vi "rszvl_core_global.vi"() -> ()   [LabVIEW 2014] (continued)
"Restricted Repeated Capabilities"="", "Help"="This attribute switches on and off the calibration info in the custom header. The custom header can be added to an exported trace file.\n\nAvailable Repeated Capabilities:\nNone\n\nRemote-control command(s):\nMMEMory:STORe:TRACe:USER:CINFo ON | OFF", "Flags"={"OPC Wait"=FALSE, "Dont check status"=FALSE, "*WAI"=FALSE}, "Check Status Callback"=""}, {"Level"=1, "Descriptive Name"="NWA Markers", "Class Only"=TRUE, "Data Type"=0, "Access"=0, "Identifier"="", "Range Table"="", "Command"="", "Read Callback"="", "Write Callback"="", "Range Callback"="", "Check Callback"="", "Rngtable Callback"="", "Coerce Callback"="", "User Callback"="", "Supported Models"="", "Instrument Options"="", "Repeated Capabilities"="", "Restricted Repeated Capabilities"="", "Help"="(1) NWA Marker State:\nThis attribute creates the marker numbered <Mk> and assigns it to trace no. <Chn>.\n\n(2) NWA Marker Stimulus:\nThis attribute defines the stimulus (in Cartesian diagrams: x-axis) value of the marker no. <Mk>, which can (but doesn't have to) be created using CALCulate<Chn>:MARKer<Mk>[:STATe] ON (attribute RSZVL_ATTR_NWA_MARKER_STATE).\n\n(3) NWA Marker Reference State:\nThis attribute creates the reference marker and assigns it to trace no. <Chn>.\n\n(4) NWA Marker Reference Stimulus:\nThis attribute defines the stimulus (in Cartesian diagrams: x-axis) value of the reference marker, which can (but doesn't have to) be displayed using CALCulate<Chn>:MARKer<Mk>:REFerence[:STATe] ON (attribute RSZVL_ATTR_NWA_MARKER_STATE). \n\n(5) NWA Delta Marker State:\nThis attribute switches the delta mode for marker <Mk> on trace no. <Chn> on or off. The marker must be created before using CALCulate<Chn>:MARKer<Mk>[:STATe] ON (attribute RSZVL_ATTR_NWA_MARKER_STATE). If the active trace contains no reference marker, the command also creates a reference marker.\n\n(6) NWA Marker Coupled:\nThis attribute couples the markers of all traces in the active setup to the markers of trace no. <Chn>, provided that they have the same sweep type (SENSe<Chn>:FUNCtion).\n\n(7) NWA Marker Mode:\nThis attribute sets marker no. <Mk> to continuous or discrete mode. The marker doesn't have to be created before (CALCulate<Chn>:MARKer<Mk>[:STATe] ON), the mode can be assigned in advance.\n\n(8) NWA Marker Fixed:\nThis attribute sets marker no. <Mk> to normal or fixed mode. The marker must be created before using CALCulate<Ch/Tr>:MARKer<Mk>[:STATe] ON (attribute RSZVL_ATTR_NWA_MARKER_STATE). \n\n(9) NWA Marker Search Tracking:\nThis attribute enables or disables the marker tracking mode for marker no. <Mk>. Tracking mode causes the active minimum/maximum or target search of the active marker to be repeated after each sweep. A marker must be created and a search mode must be active (CALCulate<Chn>:MARKer<Mk>:FUNCtion:EXECute ...) to use this attribute.\n\n(10) NWA All Markers Off:\nThis attribute removes all markers from all traces of the active setup. The removed markers remember their properties (stimulus value, format, delta mode, number) when they are restored (CALC<Chn>:MARK<Mk> ON). The marker properties are definitely lost if the associated trace is deleted. \n\n(11) NWA Marker To Center:\nThis attribute sets the center of the sweep range equal to the stimulus value of the marker <Mk> on trace no. <Chn>.\n\n(12) NWA Marker To Start Frequency:\nThis attribute sets the beginning (start) of the sweep range equal to the stimulus value of the marker <Mk> on trace no. <Chn>.\n\n(13) NWA Marker To Stop Frequency:\nThis attribute sets the end (stop) of the sweep range equal to the stimulus value of the marker <Mk> on trace no. <Chn>.\n\n(14) NWA Marker Format:\nThis attribute defines the output format for the (complex) value of marker <Mk> on trace no. <Chn>.\n\n(15) NWA Marker Search:\nThis attribute selects a search mode for marker no. <Mk> and initiates the search. The marker must be created before using CALCulate<Chn>:MARKer<Mk>[:STATe] ON (exception: bandfilter search). \n\n(16) NWA Marker Bandfilter Search Mode:\nThis attribute selects the bandfilter search mode.\n\n(17) NWA Marker Search Range:\nThis attribute assigns a search range no. <numeric_value> to marker no <Mk> and selects the search range, e.g. in order to define the start and stop values.\n\n(18) NWA Marker Search Range Start:\nThis attribute defines the start value of the search range selected with CALCulate<Chn>:MARKer<Mk>:FUNCtion:DOMain:USER (attribute RSZVL_ATTR_NWA_MARKER_SEARCH_RANGE). \n\n(19) NWA Marker Search Range Stop:\nThis attribute defines the stop value of the search range selected with CALCulate<Chn>:MARKer<Mk>:FUNCtion:DOMain:USER (attribute RSZVL_ATTR_NWA_MARKER_SEARCH_RANGE). \n\n(20) NWA Marker Target Value:\nThis attribute defines the target value for the target search of marker no. <Mk>, which can be activated using CALCulate<Chn>:MARKer<Mk>:FUCTion:EXECute TARGet (attribute RSZVL_ATTR_NWA_MARKER_SEARCH_MODE). \n\n(21) NWA Marker Bandwidth:\nThis attribute sets the bandfilter level for a bandfilter search or returns the results. The attribute is only available after a bandfilter search has been executed (CALCulate<Chn>:MARKer<Mk>:FUNCtion:EXECute BFILter).\n\n(22) NWA Marker Show Bandfilter Search Results:\nThis attribute shows or hides the bandfilter search results in the diagram area.\n\n(23) NWA Save All Markers:\nThis attribute saves the values of all markers to a ASCII file.", "Flags"={"OPC Wait"=FALSE, "Dont check status"=FALSE, "*WAI"=FALSE}, "Check Status Callback"=""}, {"Level"=2, "Descriptive Name"="NWA Marker State", "Class Only"=FALSE, "Data Type"=3, "Access"=2, "Identifier"="RSZVL_ATTR_NWA_MARKER_STATE", "Range Table"="", "Command"="CALC{Channel}:MARK{NWAMarker}:STAT", "Read Callback"="", "Write Callback"="", "Range Callback"="", "Check Callback"="", "Rngtable Callback"="", "Coerce Callback"="", "User Callback"="", "Supported Models"="", "Instrument Options"="", "Repeated Capabilities"="", "Restricted Repeated Capabilities"="", "Help"="This attribute creates the marker numbered <Mk> and assigns it to trace no. <Chn>.\n\nAvailable Repeated Capabilities:\nChannel: CH1,CH2,CH3,CH4,CH5,CH6,CH7,CH8,CH9,CH10,CH11,CH12,CH13,CH14,CH15,CH16,CH17,CH18,CH19,CH20\r\nNWAMarker: MAR1,MAR2,MAR3,MAR4,MAR5,MAR6,MAR7,MAR8,MAR9,MAR10\r\n\nRemote-control command(s):\nCALCulate<Chn>:MARKer<Mk>[:STATe] ON | OFF", "Flags"={"OPC Wait"=FALSE, "Dont check status"=FALSE, "*WAI"=FALSE}, "Check Status Callback"=""}, {"Level"=2, "Descriptive Name"="NWA Marker Stimulus", "Class Only"=FALSE, "Data Type"=1, "Access"=2, "Identifier"="RSZVL_ATTR_NWA_MARKER_X", "Range Table"="rszvl_rngNWAMarkerStimulus", "Command"="CALC{Channel}:MARK{NWAMarker}:X", "Read Callback"="", "Write Callback"="", "Range Callback"="", "Check Callback"="", "Rngtable Callback"="", "Coerce Callback"="", "User Callback"="", "Supported Models"="", "Instrument Options"="", "Repeated Capabilities"="", "Restricted Repeated Capabilities"="", "Help"="This attribute defines the stimulus (in Cartesian diagrams: x-axis) value of the marker no. <Mk>, which can (but doesn't have to) be created using CALCulate<Chn>:MARKer<Mk>[:STATe] ON (attribute RSZVL_ATTR_NWA_MARKER_STATE).\n\nAvailable Repeated Capabilities:\nChannel: CH1,CH2,CH3,CH4,CH5,CH6,CH7,CH8,CH9,CH10,CH11,CH12,CH13,CH14,CH15,CH16,CH17,CH18,CH19,CH20\r\nNWAMarker: MAR1,MAR2,MAR3,MAR4,MAR5,MAR6,MAR7,MAR8,MAR9,MAR10\r\n\nRemote-control command(s):\nCALCulate<Chn>:MARKer<Mk>:X", "Flags"={"OPC Wait"=FALSE, "Dont check status"=FALSE, "*WAI"=FALSE}, "Check Status Callback"=""}, {"Level"=2, "Descriptive Name"="NWA Marker Reference State", "Class Only"=FALSE, "Data Type"=3, "Access"=2, "Identifier"="RSZVL_ATTR_NWA_MARKER_REF_STATE", "Range Table"="", "Command"="CALC{Channel}:MARK{NWAMarker}:REF:STAT", "Read Callback"="", "Write Callback"="", "Range Callback"="", "Check Callback"="", "Rngtable Callback"="", "Coerce Callback"="", "User Callback"="", "Supported Models"="", "Instrument Options"="", "Repeated Capabilities"="", "Restricted Repeated Capabilities"="", "Help"="This attribute creates the reference marker and assigns it to trace no. <Chn>.\n\nAvailable Repeated Capabilities:\nChannel: CH1,CH2,CH3,CH4,CH5,CH6,CH7,CH8,CH9,CH10,CH11,CH12,CH13,CH14,CH15,CH16,CH17,CH18,CH19,CH20\r\nNWAMarker: MAR1,MAR2,MAR3,MAR4,MAR5,MAR6,MAR7,MAR8,MAR9,MAR10\r\n\nRemote-control command(s):\nCALCulate<Chn>:MARKer<Mk>:REFerence[:STATe] ON | OFF", "Flags"={"OPC Wait"=FALSE, "Dont check status"=FALSE, "*WAI"=FALSE}, "Check Status Callback"=""}, {"Level"=2, "Descriptive Name"="NWA Marker Reference Stimulus", "Class Only"=FALSE, "Data Type"=1, "Access"=2, "Identifier"="RSZVL_ATTR_NWA_MARKER_REF_X", "Range Table"="rszvl_rngNWAMarkerStimulus", "Command"="CALC{Channel}:MARK{NWAMarker}:REF:X", "Read Callback"="", "Write Callback"="", "Range Callback"="", "Check Callback"="", "Rngtable Callback"="", "Coerce Callback"="", "User Callback"="", "Supported Models"="", "Instrument Options"="", "Repeated Capabilities"="", "Restricted Repeated Capabilities"="", "Help"="This attribute defines the stimulus (in Cartesian diagrams: x-axis) value of the reference marker, which can (but doesn't have to) be displayed using CALCulate<Chn>:MARKer<Mk>:REFerence[:STATe] ON (attribute RSZVL_ATTR_NWA_MARKER_STATE).\n\nAvailable Repeated Capabilities:\nChannel: CH1,CH2,CH3,CH4,CH5,CH6,CH7,CH8,CH9,CH10,CH11,CH12,CH13,CH14,CH15,CH16,CH17,CH18,CH19,CH20\r\nNWAMarker: MAR1,MAR2,MAR3,MAR4,MAR5,MAR6,MAR7,MAR8,MAR9,MAR10\r\n\nRemote-control command(s):\nCALCulate<Chn>:MARKer<Mk>:REFerence:X", "Flags"={"OPC Wait"=FALSE, "Dont check status"=FALSE, "*WAI"=FALSE}, "Check Status Callback"=""}, {"Level"=2, "Descriptive Name"="NWA Marker Reference Mode", "Class Only"=FALSE, "Data Type"=0, "Access"=2, "Identifier"="RSZVL_ATTR_NWA_MARKER_REF_MODE", "Range Table"="rszvl_rngNWAMarkerMode", "Command"="CALC{Channel}:MARK{NWAMarker}:REF:MODE", "Read Callback"="", "Write Callback"="", "Range Callback"="", "Check Callback"="", "Rngtable Callback"="", "Coerce Callback"="", "User Callback"="", "Supported Models"="", "Instrument Options"="", "Repeated Capabilities"="", "Restricted Repeated Capabilities"="", "Help"="This attribute sets the reference marker to continuous or discrete mode. The marker doesn't have to be created before\n(CALCulate<Chn>:MARKer<Mk>:REFerence[:STATe] ON), the mode can be assigned in advance.\n\nAvailable Repeated Capabilities:\nChannel: CH1,CH2,CH3,CH4,CH5,CH6,CH7,CH8,CH9,CH10,CH11,CH12,CH13,CH14,CH15,CH16,CH17,CH18,CH19,CH20\r\nNWAMarker: MAR1,MAR2,MAR3,MAR4,MAR5,MAR6,MAR7,MAR8,MAR9,MAR10\r\n\nRemote-control command(s):\nCALCulate<Chn>:MARKer<Mk>:REFerence:MODE CONTinuous | DISCrete", "Flags"={"OPC Wait"=FALSE, "Dont check status"=FALSE, "*WAI"=FALSE}, "Check Status Callback"=""}, {"Level"=2, "Descriptive Name"="NWA Marker Referece Fixed", "Class Only"=FALSE, "Data Type"=0, "Access"=2, "Identifier"="RSZVL_ATTR_NWA_MARKER_REF_FIXED", "Range Table"="rszvl_rngNWAMarkerType", "Command"="CALC{Channel}:MARK{NWAMarker}:REF:TYPE", "Read Callback"="", "Write Callback"="", "Range Callback"="", "Check Callback"="", "Rngtable Callback"="", "Coerce Callback"="", "User Callback"="", "Supported Models"="", "Instrument Options"="", "Repeated Capabilities"="", "Restricted Repeated Capabilities"="", "Help"="This attribute sets the reference to normal or fixed mode. The marker must be created before using\nCALCulate<Chn>:MARKer<Mk>:REFerence[:STATe] ON.\n\nAvailable Repeated Capabilities:\nChannel: CH1,CH2,CH3,CH4,CH5,CH6,CH7,CH8,CH9,CH10,CH11,CH12,CH13,CH14,CH15,CH16,CH17,CH18,CH19,CH20\r\nNWAMarker: MAR1,MAR2,MAR3,MAR4,MAR5,MAR6,MAR7,MAR8,MAR9,MAR10\r\n\nRemote-control command(s):\nCALCulate<Chn>:MARKer<Mk>:REFerence:TYPE NORMal | FIXed", "Flags"={"OPC Wait"=FALSE, "Dont check status"=FALSE, "*WAI"=FALSE}, "Check Status Callback"=""}, {"Level"=2, "Descriptive Name"="NWA Delta Marker State", "Class Only"=FALSE, "Data Type"=3, "Access"=2, "Identifier"="RSZVL_ATTR_NWA_DELTA_MARKER_STATE", "Range Table"="", "Command"="CALC{Channel}:MARK{NWAMarker}:DELT:STAT", "Read Callback"="", "Write Callback"="", "Range Callback"="", "Check Callback"="", "Rngtable Callback"="", "Coerce Callback"="", "User Callback"="", "Supported Models"="", "Instrument Options"="", "Repeated Capabilities"="", "Restricted Repeated Capabilities"="", "Help"="This attribute switches the delta mode for marker <Mk> on trace no. <Chn> on or off. The marker must be created before using CALCulate<Chn>:MARKer<Mk>[:STATe] ON (attribute RSZVL_ATTR_NWA_MARKER_STATE). If the active trace contains no reference marker, the command also creates a reference marker.\n\nAvailable Repeated Capabilities:\nChannel: CH1,CH2,CH3,CH4,CH5,CH6,CH7,CH8,CH9,CH10,CH11,CH12,CH13,CH14,CH15,CH16,CH17,CH18,CH19,CH20\r\nNWAMarker: MAR1,MAR2,MAR3,MAR4,MAR5,MAR6,MAR7,MAR8,MAR9,MAR10\r\n\nRemote-control command(s):\nCALCulate<Chn>:MARKer<Mk>:DELTa[:STATe] ON | OFF", "Flags"={"OPC Wait"=FALSE, "Dont check status"=FALSE, "*WAI"=FALSE}, "Check Status Callback"=""}, {"Level"=2, "Descriptive Name"="NWA Marker Coupled", "Class Only"=FALSE, "Data Type"=3, "Access"=2, "Identifier"="RSZVL_ATTR_NWA_MARKER_COUPLED", "Range Table"="", "Command"="CALC{Channel}:MARK:COUP:STAT", "Read Callback"="", "Write Callback"="", "Range Callback"="", "Check Callback"="", "Rngtable Callback"="", "Coerce Callback"="", "User Callback"="", "Supported Models"="", "Instrument Options"="", "Repeated Capabilities"="", "Restricted Repeated Capabilities"="", "Help"="This attribute couples the markers of all traces in the active setup to the markers of trace no. <Chn>, provided that they have the same sweep type (SENSe<Chn>:FUNCtion).\n\nAvailable Repeated Capabilities:\nChannel: CH1,CH2,CH3,CH4,CH5,CH6,CH7,CH8,CH9,CH10,CH11,CH12,CH13,CH14,CH15,CH16,CH17,CH18,CH19,CH20\r\n\nRemote-control command(s):\nCALCulate<Chn>:MARKer<Mk>:COUPled[:STATe] ON | OFF", "Flags"={"OPC Wait"=FALSE, "Dont check status"=FALSE, "*WAI"=FALSE}, "Check Status Callback"=""}, {"Level"=2, "Descriptive Name"="NWA Marker Mode", "Class Only"=FALSE, "Data Type"=0, "Access"=2, "Identifier"="RSZVL_ATTR_NWA_MARKER_MODE", "Range Table"="rszvl_rngNWAMarkerMode", "Command"="CALC{Channel}:MARK{NWAMarker}:MODE", "Read Callback"="", "Write Callback"="", "Range Callback"="", "Check Callback"="", "Rngtable Callback"="", "Coerce Callback"="", "User Callback"="", "Supported Models"="", "Instrument Options"="", "Repeated Capabilities"="", "Restricted Repeated Capabilities"="", "Help"="This attribute sets marker no. <Mk> to continuous or discrete mode. The marker doesn't have to be created before (CALCulate<Chn>:MARKer<Mk>[:STATe] ON), the mode can be assigned in advance.\n\nAvailable Repeated Capabilities:\nChannel: CH1,CH2,CH3,CH4,CH5,CH6,CH7,CH8,CH9,CH10,CH11,CH12,CH13,CH14,CH15,CH16,CH17,CH18,CH19,CH20\r\nNWAMarker: MAR1,MAR2,MAR3,MAR4,MAR5,MAR6,MAR7,MAR8,MAR9,MAR10\r\n\nRemote-control command(s):\nCALCulate<Chn>:MARKer<Mk>:MODE CONTinuous | DISCrete", "Flags"={"OPC Wait"=FALSE, "Dont check status"=FALSE, "*WAI"=FALSE}, "Check Status Callback"=""}, {"Level"=2, "Descriptive Name"="NWA Marker Fixed", "Class Only"=FALSE, "Data Type"=0, "Access"=2, "Identifier"="RSZVL_ATTR_NWA_MARKER_TYPE", "Range Table"="rszvl_rngNWAMarkerType", "Command"="CALC{Channel}:MARK{NWAMarker}:TYPE", "Read Callback"="", "Write Callback"="", "Range Callback"="", "Check Callback"="", "Rngtable Callback"="", "Coerce Callback"="", "User Callback"="", "Supported Models"="", "Instrument Options"="", "Repeated Capabilities"="", "Restricted Repeated Capabilities"="", "Help"="This attribute sets marker no. <Mk> to normal or fixed mode. The marker must be created before using CALCulate<Ch/Tr>:MARKer<Mk>[:STATe] ON (attribute RSZVL_ATTR_NWA_MARKER_STATE).\n\nAvailable Repeated Capabilities:\nChannel: CH1,CH2,CH3,CH4,CH5,CH6,CH7,CH8,CH9,CH10,CH11,CH12,CH13,CH14,CH15,CH16,CH17,CH18,CH19,CH20\r\nNWAMarker: MAR1,MAR2,MAR3,MAR4,MAR5,MAR6,MAR7,MAR8,MAR9,MAR10\r\n\nRemote-control command(s):\nCALCulate<Chn>:MARKer<Mk>:TYPE NORMal | FIXed", "Flags"={"OPC Wait"=FALSE, "Dont check status"=FALSE, "*WAI"=FALSE}, "Check Status Callback"=""}, {"Level"=2, "Descriptive Name"="NWA Marker Search Tracking", "Class Only"=FALSE, "Data Type"=3, "Access"=2, "Identifier"="RSZVL_ATTR_NWA_MARKER_SEARCH_TRACKING", "Range Table"="", "Command"="CALC{Channel}:MARK{NWAMarker}:SEAR:TRAC", "Read Callback"="", "Write Callback"="", "Range Callback"="", "Check Callback"="", "Rngtable Callback"="", "Coerce Callback"="", "User Callback"="", "Supported Models"="", "Instrument Options"="", "Repeated Capabilities"="", "Restricted Repeated Capabilities"="", "Help"="This attribute enables or disables the marker tracking mode for marker no. <Mk>. Tracking mode causes the active minimum/maximum or target search of the active marker to be repeated after each sweep. A marker must be created and a search mode must be active (CALCulate<Chn>:MARKer<Mk>:FUNCtion:EXECute ...) to use this attribute.\n\nAvailable Repeated Capabilities:\nChannel: CH1,CH2,CH3,CH4,CH5,CH6,CH7,CH8,CH9,CH10,CH11,CH12,CH13,CH14,CH15,CH16,CH17,CH18,CH19,CH20\r\nNWAMarker: MAR1,MAR2,MAR3,MAR4,MAR5,MAR6,MAR7,MAR8,MAR9,MAR10\r\n\nRemote-control command(s):\nCALCulate<Chn>:MARKer<Mk>:SEARch:TRACking ON | OFF", "Flags"={"OPC Wait"=FALSE, "Dont check status"=FALSE, "*WAI"=FALSE}, "Check Status Callback"=""}, {"Level"=2, "Descriptive Name"="NWA All Markers Off", "Class Only"=FALSE, "Data Type"=4, "Access"=1, "Identifier"="RSZVL_ATTR_NWA_MARKER_AOFF", "Range Table"="", "Command"="CALC{Channel}:MARK:AOFF", "Read Callback"="", "Write Callback"="", "Range Callback"="", "Check Callback"="", "Rngtable Callback"="", "Coerce Callback"="", "User Callback"="", "Supported Models"="", "Instrument Options"="", "Repeated Capabilities"="", "Restricted Repeated Capabilities"="", "Help"="This attribute removes all markers from all traces of the active setup. The removed markers remember their properties (stimulus value, format, delta mode, number) when they are restored (CALC<Chn>:MARK<Mk> ON). The marker properties are definitely lost if the associated trace is deleted.\n\nAvailable Repeated Capabilities:\nChannel: CH1,CH2,CH3,CH4,CH5,CH6,CH7,CH8,CH9,CH10,CH11,CH12,CH13,CH14,CH15,CH16,CH17,CH18,CH19,CH20\r\n\nRemote-control command(s):\nCALCulate<Chn>:MARKer<Mk>:AOFF", "Flags"={"OPC Wait"=FALSE, "Dont check status"=FALSE, "*WAI"=FALSE}, "Check Status Callback"=""}, {"Level"=2, "Descriptive Name"="NWA Marker To Center", "Class Only"=FALSE, "Data Type"=4, "Access"=1, "Identifier"="RSZVL_ATTR_NWA_MARKER_TO_CENTER", "Range Table"="", "Command"="CALC{Channel}:MARK{NWAMarker}:FUNC:CENT", "Read Callback"="", "Write Callback"="", "Range Callback"="", "Check Callback"="", "Rngtable Callback"="", "Coerce Callback"="", "User Callback"="", "Supported Models"="", "Instrument Options"="", "Repeated Capabilities"="", "Restricted Repeated Capabilities"="", "Help"="This attribute sets the center of the sweep range equal to the stimulus value of the marker <Mk> on trace no. <Chn>.\n\nAvailable Repeated Capabilities:\nChannel: CH1,CH2,CH3,CH4,CH5,CH6,CH7,CH8,CH9,CH10,CH11,CH12,CH13,CH14,CH15,CH16,CH17,CH18,CH19,CH20\r\nNWAMarker: MAR1,MAR2,MAR3,MAR4,MAR5,MAR6,MAR7,MAR8,MAR9,MAR10\r\n\nRemote-control command(s):\nCALCulate<Chn>:MARKer<Mk>:FUNCtion:CENTer", "Flags"={"OPC Wait"=FALSE, "Dont check status"=FALSE, "*WAI"=FALSE}, "Check Status Callback"=""}, {"Level"=2, "Descriptive Name"="NWA Marker To Start Frequency", "Class Only"=FALSE, "Data Type"=4, "Access"=1, "Identifier"="RSZVL_ATTR_NWA_MARKER_TO_START", "Range Table"="", "Command"="CALC{Channel}:MARK{NWAMarker}:FUNC:STAR", "Read Callback"="", "Write Callback"="", "Range Callback"="", "Check Callback"="", "Rngtable Callback"="", "Coerce Callback"="", "User Callback"="", "Supported Models"="", "Instrument Options"="", "Repeated Capabilities"="", "Restricted Repeated Capabilities"="", "Help"="This attribute sets the beginning (start) of the sweep range equal to the stimulus value of the marker <Mk> on trace no. <Chn>.\n\nAvailable Repeated Capabilities:\nChannel: CH1,CH2,CH3,CH4,CH5,CH6,CH7,CH8,CH9,CH10,CH11,CH12,CH13,CH14,CH15,CH16,CH17,CH18,CH19,CH20\r\nNWAMarker: MAR1,MAR2,MAR3,MAR4,MAR5,MAR6,MAR7,MAR8,MAR9,MAR10\r\n\nRemote-control command(s):\nCALCulate<Chn>:MARKer<Mk>:FUNCtion:STARt", "Flags"={"OPC Wait"=FALSE, "Dont check status"=FALSE, "*WAI"=FALSE}, "Check Status Callback"=""}, {"Level"=2, "Descriptive Name"="NWA Marker To Stop Frequency", "Class Only"=FALSE, "Data Type"=4, "Access"=1, "Identifier"="RSZVL_ATTR_NWA_MARKER_TO_STOP", "Range Table"="", "Command"="CALC{Channel}:MARK{NWAMarker}:FUNC:STOP", "Read Callback"="", "Write Callback"="", "Range Callback"="", "Check Callback"="", "Rngtable Callback"="", "Coerce Callback"="", "User Callback"="", "Supported Models"="", "Instrument Options"="", "Repeated Capabilities"="", "Restricted Repeated Capabilities"="", "Help"="This attribute sets the end (stop) of the sweep range equal to the stimulus value of the marker <Mk> on trace no. <Chn>.\n\nAvailable Repeated Capabilities:\nChannel: CH1,CH2,CH3,CH4,CH5,CH6,CH7,CH8,CH9,CH10,CH11,CH12,CH13,CH14,CH15,CH16,CH17,CH18,CH19,CH20\r\nNWAMarker: MAR1,MAR2,MAR3,MAR4,MAR5,MAR6,MAR7,MAR8,MAR9,MAR10\r\n\nRemote-control command(s):\nCALCulate<Chn>:MARKer<Mk>:FUNCtion:STOP", "Flags"={"OPC Wait"=FALSE, "Dont check status"=FALSE, "*WAI"=FALSE}, "Check Status Callback"=""}, {"Level"=2, "Descriptive Name"="NWA Marker Format", "Class Only"=FALSE, "Data Type"=0, "Access"=2, "Identifier"="RSZVL_ATTR_NWA_MARKER_FORMAT", "Range Table"="rszvl_rngNWAMarkerFormat", "Command"="CALC{Channel}:MARK{NWAMarker}:FORM", "Read Callback"="", "Write Callback"="", "Range Callback"="", "Check Callback"="", "Rngtable Callback"="", "Coerce Callback"="", "User Callback"="", "Supported Models"="", "Instrument Options"="", "Repeated Capabilities"="", "Restricted Repeated Capabilities"="", "Help"="This attribute defines the output format for the (complex) value of marker <Mk> on trace no. <Chn>.\n\nAvailable Repeated Capabilities:\nChannel: CH1,CH2,CH3,CH4,CH5,CH6,CH7,CH8,CH9,CH10,CH11,CH12,CH13,CH14,CH15,CH16,CH17,CH18,CH19,CH20\r\nNWAMarker: MAR1,MAR2,MAR3,MAR4,MAR5,MAR6,MAR7,MAR8,MAR9,MAR10\r\n\nRemote-control command(s):\nCALCulate<Chn>:MARKer<Mk>:FORMat MLINear | MLOGarithmic | PHASe | POLar | GDELay | REAL | IMAGinary | SWR | LINPhase | LOGPhase | IMPedance | ADMittance", "Flags"={"OPC Wait"=FALSE, "Dont check status"=FALSE, "*WAI"=FALSE}, "Check Status Callback"=""}, {"Level"=2, "Descriptive Name"="NWA Marker Search", "Class Only"=FALSE, "Data Type"=0, "Access"=1, "Identifier"="RSZVL_ATTR_NWA_MARKER_SEARCH_MODE", "Range Table"="rszvl_rngNWAMarkerSearch", "Command"="CALC{Channel}:MARK{NWAMarker}:FUNC:EXEC", "Read Callback"="", "Write Callback"="", "Range Callback"="", "Check Callback"="", "Rngtable Callback"="", "Coerce Callback"="", "User Callback"="", "Supported Models"="", "Instrument Options"="", "Repeated Capabilities"="", "Restricted Repeated Capabilities"="", "Help"="This attribute selects a search mode for marker no. <Mk> and initiates the search. The marker must be created before using CALCulate<Chn>:MARKer<Mk>[:STATe] ON (exception: bandfilter search).\n\nAvailable Repeated Capabilities:\nChannel: CH1,CH2,CH3,CH4,CH5,CH6,CH7,CH8,CH9,CH10,CH11,CH12,CH13,CH14,CH15,CH16,CH17,CH18,CH19,CH20\r\nNWAMarker: MAR1,MAR2,MAR3,MAR4,MAR5,MAR6,MAR7,MAR8,MAR9,MAR10\r\n\nRemote-control command(s):\nCALCulate<Chn>:MARKer<Mk>:FUNCtion:EXECute MAXimum | MINimum | RPEak | LPEak | NPEak | TARGet | LTARget | RTARget | BFILter", "Flags"={"OPC Wait"=FALSE, "Dont check status"=FALSE, "*WAI"=FALSE}, "Check Status Callback"=""}, {"Level"=2, "Descriptive Name"="NWA Marker Bandfilter Search Mode", "Class Only"=FALSE, "Data Type"=0, "Access"=2, "Identifier"="RSZVL_ATTR_NWA_MARKER_BFILTER_SEARCH_MODE", "Range Table"="rszvl_rngNWAMarkerBFilterSearchMode", "Command"="CALC{Channel}:MARK:FUNC:BWID:MODE", "Read Callback"="", "Write Callback"="", "Range Callback"="", "Check Callback"="", "Rngtable Callback"="", "Coerce Callback"="", "User Callback"="", "Supported Models"="", "Instrument Options"="", "Repeated Capabilities"="", "Restricted Repeated Capabilities"="", "Help"="This attribute selects the bandfilter search mode.\n\nAvailable Repeated Capabilities:\nChannel: CH1,CH2,CH3,CH4,CH5,CH6,CH7,CH8,CH9,CH10,CH11,CH12,CH13,CH14,CH15,CH16,CH17,CH18,CH19,CH20\r\n\nRemote-control command(s):\nCALCulate<Chn>:MARKer<Mk>:FUNCtion:BWIDth:MODE BPASs | BSTop | BPRMarker | BSRMarker", "Flags"={"OPC Wait"=FALSE, "Dont check status"=FALSE, "*WAI"=FALSE}, "Check Status Callback"=""}, {"Level"=2, "Descriptive Name"="NWA Marker Search Range", "Class Only"=FALSE, "Data Type"=0, "Access"=2, "Identifier"="RSZVL_ATTR_NWA_MARKER_SEARCH_RANGE", "Range Table"="rszvl_rngNWAMarkerSearchRange", "Command"="CALC{Channel}:MARK{NWAMarker}:FUNC:DOM:USER", "Read Callback"="", "Write Callback"="", "Range Callback"="", "Check Callback"="", "Rngtable Callback"="", "Coerce Callback"="", "User Callback"="", "Supported Models"="", "Instrument Options"="", "Repeated Capabilities"="", "Restricted Repeated Capabilities"="", "Help"="This attribute assigns a search range no. <numeric_value> to marker no <Mk> and selects the search range, e.g. in order to define the start and stop values.\n\nAvailable Repeated Capabilities:\nChannel: CH1,CH2,CH3,CH4,CH5,CH6,CH7,CH8,CH9,CH10,CH11,CH12,CH13,CH14,CH15,CH16,CH17,CH18,CH19,CH20\r\nNWAMarker: MAR1,MAR2,MAR3,MAR4,MAR5,MAR6,MAR7,MAR8,MAR9,MAR10\r\n\nRemote-control command(s):\nCALCulate<Chn>:MARKer<Mk>:FUNCtion:DOMain:USER", "Flags"={"OPC Wait"=FALSE, "Dont check status"=FALSE, "*WAI"=FALSE}, "Check Status Callback"=""}, {"Level"=2, "Descriptive Name"="NWA Marker Search Range Start", "Class Only"=FALSE, "Data Type"=1, "Access"=2, "Identifier"="RSZVL_ATTR_NWA_MARKER_SEARCH_RANGE_START", "Range Table"="", "Command"="CALC{Channel}:MARK{NWAMarker}:FUNC:DOM:USER:STAR", "Read Callback"="", "Write Callback"="", "Range Callback"="", "Check Callback"="", "Rngtable Callback"="", "Coerce Callback"="", "User Callback"="", "Supported Models"="", "Instrument Options"="", "Repeated Capabilities"="", "Restricted Repeated Capabilities"="", "Help"="This attribute defines the start value of the search range selected with CALCulate<Chn>:MARKer<Mk>:FUNCtion:DOMain:USER (attribute RSZVL_ATTR_NWA_MARKER_SEARCH_RANGE).\n\nAvailable Repeated Capabilities:\nChannel: CH1,CH2,CH3,CH4,CH5,CH6,CH7,CH8,CH9,CH10,CH11,CH12,CH13,CH14,CH15,CH16,CH17,CH18,CH19,CH20\r\nNWAMarker: MAR1,MAR2,MAR3,MAR4,MAR5,MAR6,MAR7,MAR8,MAR9,MAR10\r\n\nRemote-control command(s):\nCALCulate<Chn>:MARKer<Mk>:FUNCtion:DOMain:USER:STARt", "Flags"={"OPC Wait"=FALSE, "Dont check status"=FALSE, "*WAI"=FALSE}, "Check Status Callback"=""}, {"Level"=2, "Descriptive Name"="NWA Marker Search Range Stop", "Class Only"=FALSE, "Data Type"=1, "Access"=2, "Identifier"="RSZVL_ATTR_NWA_MARKER_SEARCH_RANGE_STOP", "Range Table"="", "Command"="CALC{Channel}:MARK{NWAMarker}:FUNC:DOM:USER:STOP", "Read Callback"="", "Write Callback"="", "Range Callback"="", "Check Callback"="", "Rngtable Callback"="", "Coerce Callback"="", "User Callback"="", "Supported Models"="", "Instrument Options"="", "Repeated Capabilities"="", "Restricted Repeated Capabilities"="", "Help"="This attribute defines the stop value of the search range selected with CALCulate<Chn>:MARKer<Mk>:FUNCtion:DOMain:USER (attribute RSZVL_ATTR_NWA_MARKER_SEARCH_RANGE).\n\nAvailable Repeated Capabilities:\nChannel: CH1,CH2,CH3,CH4,CH5,CH6,CH7,CH8,CH9,CH10,CH11,CH12,CH13,CH14,CH15,CH16,CH17,CH18,CH19,CH20\r\nNWAMarker: MAR1,MAR2,MAR3,MAR4,MAR5,MAR6,MAR7,MAR8,MAR9,MAR10\r\n\nRemote-control command(s):\nCALCulate<Chn>:MARKer<Mk>:FUNCtion:DOMain:USER:STOP", "Flags"={"OPC Wait"=FALSE, "Dont check status"=FALSE, "*WAI"=FALSE}, "Check Status Callback"=""}, {"Level"=2, "Descriptive Name"="NWA Marker Target Value", "Class Only"=FALSE, "Data Type"=1, "Access"=2, "Identifier"="RSZVL_ATTR_NWA_MARKER_TARGET_VALUE", "Range Table"="", "Command"="CALC{Channel}:MARK{NWAMarker}:TARG", "Read Callback"="", "Write Callback"="", "Range Callback"="", "Check Callback"="", "Rngtable Callback"="", "Coerce Callback"="", "User Callback"="", "Supported Models"="", "Instrument Options"="", "Repeated Capabilities"="", "Restricted Repeated Capabilities"="", "Help"="This attribute defines the target value for the target search of marker no. <Mk>, which can be activated using CALCulate<Chn>:MARKer<Mk>:FUCTion:EXECute TARGet (attribute RSZVL_ATTR_NWA_MARKER_SEARCH_MODE).\n\nAvailable Repeated Capabilities:\nChannel: CH1,CH2,CH3,CH4,CH5,CH6,CH7,CH8,CH9,CH10,CH11,CH12,CH13,CH14,CH15,CH16,CH17,CH18,CH19,CH20\r\nNWAMarker: MAR1,MAR2,MAR3,MAR4,MAR5,MAR6,MAR7,MAR8,MAR9,MAR10\r\n\nRemote-control command(s):\nCALCulate<Chn>:MARKer<Mk>:TARGet", "Flags"={"OPC Wait"=FALSE, "Dont check status"=FALSE, "*WAI"=FALSE}, "Check Status Callback"=""}, {"Level"=2, "Descriptive Name"="NWA Marker Bandwidth", "Class Only"=FALSE, "Data Type"=1, "Access"=1, "Identifier"="RSZVL_ATTR_NWA_MARKER_BANDWIDTH", "Range Table"="rszvl_rngMarkerNdBDown", "Command"="CALC{Channel}:MARK:BWID", "Read Callback"="", "Write Callback"="", "Range Callback"="", "Check Callback"="", "Rngtable Callback"="", "Coerce Callback"="", "User Callback"="", "Supported Models"="", "Instrument Options"="", "Repeated Capabilities"="", "Restricted Repeated Capabilities"="", "Help"="This attribute sets the bandfilter level for a bandfilter search or returns the results. The attribute is only available after a bandfilter search has been executed (CALCulate<Chn>:MARKer<Mk>:FUNCtion:EXECute BFILter).\n\nAvailable Repeated Capabilities:\nChannel: CH1,CH2,CH3,CH4,CH5,CH6,CH7,CH8,CH9,CH10,CH11,CH12,CH13,CH14,CH15,CH16,CH17,CH18,CH19,CH20\r\n\nRemote-control command(s):\nCALCulate<Chn>:MARKer<Mk>:BWIDth", "Flags"={"OPC Wait"=FALSE, "Dont check status"=FALSE, "*WAI"=FALSE}, "Check Status Callback"=""}, {"Level"=2, "Descriptive Name"="NWA Marker Show Bandfilter Search Results", "Class Only"=FALSE, "Data Type"=3, "Access"=2, "Identifier"="RSZVL_ATTR_NWA_MARKER_BFILT_SEARCH_RESULTS", "Range Table"="", "Command"="CALC{Channel}:MARK:SEAR:BFIL:RES:STAT", "Read Callback"="", "Write Callback"="", "Range Callback"="", "Check Callback"="", "Rngtable Callback"="", "Coerce Callback"="", "User Callback"="", "Supported Models"="", "Instrument Options"="", "Repeated Capabilities"="", "Restricted Repeated Capabilities"="", "Help"="This attribute shows or hides the bandfilter search results in the diagram area.\n\nAvailable Repeated Capabilities:\nChannel: CH1,CH2,CH3,CH4,CH5,CH6,CH7,CH8,CH9,CH10,CH11,CH12,CH13,CH14,CH15,CH16,CH17,CH18,CH19,CH20\r\n\nRemote-control command(s):\nCALCulate<Chn>:MARKer<Mk>:SEARch:BFILter:RESult[:STATe] ON | OFF", "Flags"={"OPC Wait"=FALSE, "Dont check status"=FALSE, "*WAI"=FALSE}, "Check Status Callback"=""}, {"Level"=2, "Descriptive Name"="NWA Save All Markers", "Class Only"=FALSE, "Data Type"=2, "Access"=1, "Identifier"="RSZVL_ATTR_NWA_SAVE_ALL_MARKERS", "Range Table"="", "Command"="MMEM:STOR:MARK", "Read Callback"="", "Write Callback"="rszvl_quotedString_WriteCallback.vi", "Range Callback"="", "Check Callback"="", "Rngtable Callback"="", "Coerce Callback"="", "User Callback"="", "Supported Models"="", "Instrument Options"="", "Repeated Capabilities"="", "Restricted Repeated Capabilities"="", "Help"="This attribute saves the values of all markers to a ASCII file.\n\nAvailable Repeated Capabilities:\nNone\n\nRemote-control command(s):\nMMEMory:STORe:MARKer '<file_name>'", "Flags"={"OPC Wait"=FALSE, "Dont check status"=FALSE, "*WAI"=FALSE}, "Check Status Callback"=""}, {"Level"=1, "Descriptive Name"="NWA Limit Lines", "Class Only"=TRUE, "Data Type"=0, "Access"=0, "Identifier"="", "Range Table"="", "Command"="", "Read Callback"="", "Write Callback"="", "Range Callback"="", "Check Callback"="", "Rngtable Callback"="", "Coerce Callback"="", "User Callback"="", "Supported Models"="", "Instrument Options"="", "Repeated Capabilities"="", "Restricted Repeated Capabilities"="", "Help"="(1) NWA Limit Display State:\nThis attribute displays or hides the entire limit line (including all segments) associated to the active trace.\n\n(2) NWA Limit State:\nThis attribute switches the limit check (including upper and lower limits) on or off.\n\n(3) NWA Limit Lower State:\nThis attribute switches the lower limit check on or off. Lower limit line segments are assigned even numbers.\n\n(4) NWA Limit Upper State:\nThis attribute switches the upper limit check on or off. Upper limit line segments are assigned odd numbers.\n\n(5) NWA Limit Response Domain Complex Units:\nThis attribute deletes the existing limit line and (re-)defines the physical units of the response values of the limit line. \n\n(6) NWA Limit Response Domain Format Units:\nThis attribute deletes the existing limit line and (re-)defines the physical units of the response values of the limit line.\n\n(7) NWA Limit Response Domain Spacing Units:\nThis attribute deletes the existing limit line and (re-)defines the physical units of the response values of the limit line.\n\n(8) NWA Display Line State:\nThis attribute switches the horizontal line on or off.\n\n(9) NWA Display Line Position:\nThis attribute defines the position (response value) of the horizontal line.\n\n(10) NWA Limit Segment Type:\nThis attribute selects the limit line type for a limit line segment. This can be done before or after defining the stimulus and response values of the segment, however, a segment must be created first.\n\n(11) NWA Limit Segment Stimulus Start:\nThis attribute changes the start stimulus value (i.e. the largest or smallest stimulus value) of a limit line segment. A segment must be created first.\n\n(12) NWa Limit Segment Stimulus Stop:\nThis attribute changes the stop stimulus value (i.e. the largest or smallest stimulus value) of a limit line segment. A segment must be created first.\n\n(13) NWA Limit Segment Response Start:\nThis attribute changes the start response value (i.e. the response value assigned to the start stimulus value) of a limit line segment. A segment must be created first.\n\n(14) NWA Limit Segment Response Stop:\nThis attribute changes the stop response value (i.e. the response value assigned to the stop stimulus value) of a limit line segment. A segment must be created first.\n\n(15) NWA Limit Segment Stimulus Shift:\nThis attribute shifts the limit line in horizontal direction.\n\n(16) NWA Limit Segment Lower Shift:\nThis attribute shifts all lower and upper limit line segments assigned to the active trace in vertical direction.\n\n(17) NWA Limit Segment Upper Shift:\nThis attribute shifts all lower and upper limit line segments assigned to the active trace in vertical direction.\n\n(18) NWA Limit Delete All Segments:\nThis attribute deletes all limit line segments.", "Flags"={"OPC Wait"=FALSE, "Dont check status"=FALSE, "*WAI"=FALSE}, "Check Status Callback"=""}, {"Level"=2, "Descriptive Name"="NWA Limit Display State", "Class Only"=FALSE, "Data Type"=3, "Access"=2, "Identifier"="RSZVL_ATTR_NWA_LIMIT_DISPLAY_STATE", "Range Table"="", "Command"="CALC{Channel}:LIM:DISP:STAT", "Read Callback"="", "Write Callback"="", "Range Callback"="", "Check Callback"="", "Rngtable Callback"="", "Coerce Callback"="", "User Callback"="", "Supported Models"="", "Instrument Options"="", "Repeated Capabilities"="", "Restricted Repeated Capabilities"="", "Help"="This attribute displays or hides the entire limit line (including all segments) associated to the active trace.\n\nAvailable Repeated Capabilities:\nChannel: CH1,CH2,CH3,CH4,CH5,CH6,CH7,CH8,CH9,CH10,CH11,CH12,CH13,CH14,CH15,CH16,CH17,CH18,CH19,CH20\r\n\nRemote-control command(s):\nCALCulate<Chn>:LIMit:DISPlay[:STATe] ON | OFF", "Flags"={"OPC Wait"=FALSE, "Dont check status"=FALSE, "*WAI"=FALSE}, "Check Status Callback"=""}, {"Level"=2, "Descriptive Name"="NWA Limit State", "Class Only"=FALSE, "Data Type"=3, "Access"=2, "Identifier"="RSZVL_ATTR_NWA_LIMIT_STATE", "Range Table"="", "Command"="CALC{Channel}:LIM:STAT", "Read Callback"="", "Write Callback"="", "Range Callback"="", "Check Callback"="", "Rngtable Callback"="", "Coerce Callback"="", "User Callback"="", "Supported Models"="", "Instrument Options"="", "Repeated Capabilities"="", "Restricted Repeated Capabilities"="", "Help"="This attribute switches the limit check (including upper and lower limits) on or off.\n\nAvailable Repeated Capabilities:\nChannel: CH1,CH2,CH3,CH4,CH5,CH6,CH7,CH8,CH9,CH10,CH11,CH12,CH13,CH14,CH15,CH16,CH17,CH18,CH19,CH20\r\n\nRemote-control command(s):\nCALCulate<Chn>:LIMit:STATe ON | OFF", "Flags"={"OPC Wait"=FALSE, "Dont check status"=FALSE, "*WAI"=FALSE}, "Check Status Callback"=""}, {"Level"=2, "Descriptive Name"="NWA Limit Lower State", "Class Only"=FALSE, "Data Type"=3, "Access"=2, "Identifier"="RSZVL_ATTR_NWA_LIMIT_LOWER_STATE", "Range Table"="", "Command"="CALC{Channel}:LIM:LOW:STAT", "Read Callback"="", "Write Callback"="", "Range Callback"="", "Check Callback"="", "Rngtable Callback"="", "Coerce Callback"="", "User Callback"="", "Supported Models"="", "Instrument Options"="", "Repeated Capabilities"="", "Restricted Repeated Capabilities"="", "Help"="This attribute switches the lower limit check on or off. Lower limit line segments are assigned even numbers.\n\nAvailable Repeated Capabilities:\nChannel: CH1,CH2,CH3,CH4,CH5,CH6,CH7,CH8,CH9,CH10,CH11,CH12,CH13,CH14,CH15,CH16,CH17,CH18,CH19,CH20\r\n\nRemote-control command(s):\nCALCulate<Chn>:LIMit:LOWer:STATe ON | OFF", "Flags"={"OPC Wait"=FALSE, "Dont check status"=FALSE, "*WAI"=FALSE}, "Check Status Callback"=""}, {"Level"=2, "Descriptive Name"="NWA Limit Upper State", "Class Only"=FALSE, "Data Type"=3, "Access"=2, "Identifier"="RSZVL_ATTR_NWA_LIMIT_UPPER_STATE", "Range Table"="", "Command"="CALC{Channel}:LIM:UPP:STAT", "Read Callback"="", "Write Callback"="", "Range Callback"="", "Check Callback"="", "Rngtable Callback"="", "Coerce Callback"="", "User Callback"="", "Supported Models"="", "Instrument Options"="", "Repeated Capabilities"="", "Restricted Repeated Capabilities"="", "Help"="This attribute switches the upper limit check on or off. Upper limit line segments are assigned odd numbers.\n\nAvailable Repeated Capabilities:\nChannel: CH1,CH2,CH3,CH4,CH5,CH6,CH7,CH8,CH9,CH10,CH11,CH12,CH13,CH14,CH15,CH16,CH17,CH18,CH19,CH20\r\n\nRemote-control command(s):\nCALCulate<Chn>:LIMit:UPPer:STATe ON | OFF", "Flags"={"OPC Wait"=FALSE, "Dont check status"=FALSE, "*WAI"=FALSE}, "Check Status Callback"=""}, {"Level"=2, "Descriptive Name"="NWA Limit Response Domain Complex Units", "Class Only"=FALSE, "Data Type"=0, "Access"=1, "Identifier"="RSZVL_ATTR_NWA_LIMIT_RDOM_COMPLEX", "Range Table"="rszvl_rngNWALimitRDOMComplex", "Command"="CALC{Channel}:LIM:RDOM:COMP", "Read Callback"="", "Write Callback"="", "Range Callback"="", "Check Callback"="", "Rngtable Callback"="", "Coerce Callback"="", "User Callback"="", "Supported Models"="", "Instrument Options"="", "Repeated Capabilities"="", "Restricted Repeated Capabilities"="", "Help"="This attribute deletes the existing limit line and (re-)defines the physical units of the response values of the limit line.\n\nAvailable Repeated Capabilities:\nChannel: CH1,CH2,CH3,CH4,CH5,CH6,CH7,CH8,CH9,CH10,CH11,CH12,CH13,CH14,CH15,CH16,CH17,CH18,CH19,CH20\r\n\nRemote-control command(s):\nCALCulate<Chn>:LIMit:RDOMain:COMPlex S | SINV | Y | Z | YREL | ZREL", "Flags"={"OPC Wait"=FALSE, "Dont check status"=FALSE, "*WAI"=FALSE}, "Check Status Callback"=""}, {"Level"=2, "Descriptive Name"="NWA Limit Response Domain Format Units", "Class Only"=FALSE, "Data Type"=0, "Access"=1, "Identifier"="RSZVL_ATTR_NWA_LIMIT_RDOM_FORMAT", "Range Table"="rszvl_rngNWALimitRDOMFormat", "Command"="CALC{Channel}:LIM:RDOM:FORM", "Read Callback"="", "Write Callback"="", "Range Callback"="", "Check Callback"="", "Rngtable Callback"="", "Coerce Callback"="", "User Callback"="", "Supported Models"="", "Instrument Options"="", 
